vi "Indicate Capillary Line.vi"(8 "error in (no error)":errorcluster, 11 "Capillary in":refnum<class "Capillary.lvclass">) -> (0 "error out":errorcluster, 3 "Capillary out":refnum<class "Capillary.lvclass">)   [LabVIEW 2015, in "AMS UI.lvlib" / "Capillary.lvclass"]
uses:
  Capillary.lvclass
  Capillary.lvclass/Capillary.ctl
  subs/Sample/Sample.lvclass/Sample.ctl
  subs/Sample/Sample.lvclass
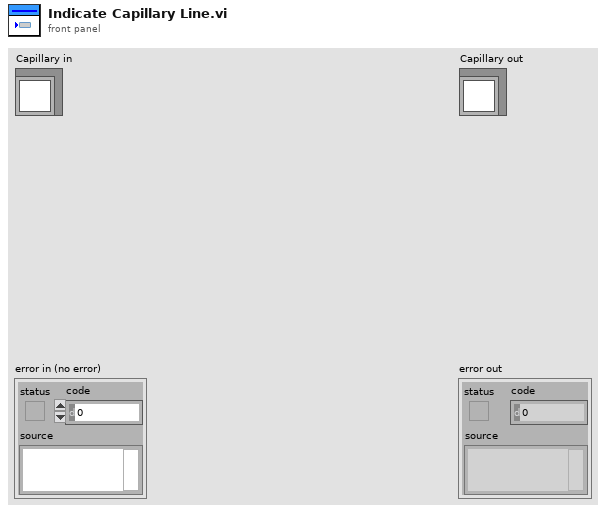
[diagram p1: front panel]
types:
  T1 = typedef "Sample Container.ctl" = cluster{"Sample In":refnum<k21>, "Sample Name":refnum<k21>, "Ti Cathode":refnum<k21>, "SampleQ":refnum<queue>}
  T2 = typedef "FP Control Refs Cluster.ctl" = cluster{"Liquid N Valve References":T3, "Main Line Valve Refs":T4, "Transfer Line Container":refnum<vi>, "Storage Containers":refnum<vi>[], "Sample Refs":T5, "Syringe Ctrl Refs ":T6, "Baratrons Chart":refnum<vi>, "Capillary Container":refnum<vi>, "Preparation Container":refnum<vi>, "Monkey Mode":refnum<vi>}
  T3 = typedef "Liquid N Valve Ref Cluster.ctl" = cluster{"Cold Bath H2O HV 100":refnum<vi>, "Cold Bath Cleaning HV 101":refnum<vi>, "Cold Bath Storage 1 HV 102":refnum<vi>, "Cold Bath Storage 2 HV 103":refnum<vi>, "Cold Bath Storage 3 HV 104":refnum<vi>, "Cold Bath Storage 4 HV 105":refnum<vi>, "Cold Bath Syringe HV 106":refnum<vi>, "Liquid N Master Valve HV 107":refnum<vi>}
  T4 = typedef "Main Line Valve Ref Cluster.ctl" = cluster{"Turbo Valve DV313":refnum<vi>, "Prep Line Valve 0 DV300":refnum<vi>, "Storage Valves":refnum<vi>[]}
  T5 = typedef "Sample Valve Refs.ctl" = cluster{"Valves":cluster{"Sample 5 DV318":refnum<vi>, "Sample 4 DV317":refnum<vi>, "Sample 3 DV316":refnum<vi>, "Sample 2 DV315":refnum<vi>, "Sample 1 DV314":refnum<vi>}, "Lines":cluster{"Sample 1":refnum<vi>, "Sample 2":refnum<vi>, "Sample 3":refnum<vi>, "Sample 4":refnum<vi>, "Sample 5":refnum<vi>}}
  T6 = typedef "Syringe Ctrl Refs.ctl" = cluster{"Syringe Home":refnum<vi>, "Syringe Freeze":refnum<vi>, "Syringe TC":refnum<vi>, "Syringe Container":refnum<vi>}
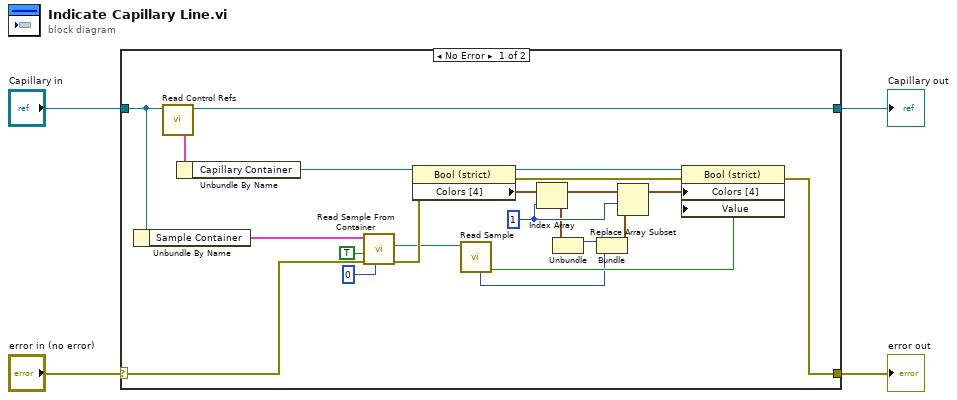
[diagram p0: block diagram]
diagram:
  n1 = case shown="No Error" "error in (no error)" {
    selector: "error in (no error)" -> [w21 w27]
    tunnel: [w5 w27] -> w2
    tunnel: [w25 w26] -> w1
    tunnel: "Capillary in" -> [w23 w26]
    frame No Error {
      w16 = 1 ("index")
      n2 = Unbundle By Name(w23) -> ("Sample Container"=w22:T1)
      n3 = call-dynamic "Read Control Refs.vi"("AMS Gas Actor in"=w23) -> ("Control Refs"=w24:T2, "AMS Gas Actor out"=w25:refnum<class "Capillary.lvclass">)  [unwired: 9 in]
      n4 = Unbundle By Name(w24) -> ("Capillary Container"=w20:refnum<vi>)
      n5 = call "Read Sample From Container.vi"("Queue timeout in ms (-1)"=0, "error in (no error)"=w21, "Read from SHV (F)"=TRUE, "Container"=w22) -> ("error out"=w11:errorcluster, "Sample out"=w10:refnum<class "Sample.lvclass">)  [unwired: 3 in, 3 out]
      n6 = property class="Bool (strict)"(reference=w20, error in=w11) -> (reference out=w19:refnum<vi>, error out=w18:errorcluster, "Colors [4]"=w17:cluster{u32, u32}[])
      n7 = call "Read Sample.vi"("Sample in"=w10) -> ("Sample In"=w9:bool, "Color"=w8:u32)  [unwired: 6 in, 3 out]
      n8 = Index Array(array=w17, index=w16) -> (element=w12:cluster{u32, u32})
      n9 = Unbundle(w12) -> (w13:u32)  [unwired: 1 out]
      n10 = Bundle(w13, "Color"=w8) -> (w15:cluster{u32, "Color":u32})  [unwired: 1 in]
      n11 = Replace Array Subset(array=w17, new element=w15, index=w16) -> (w14:cluster{u32, u32}[])
      n12 = property class="Bool (strict)"(reference=w19, error in=w18, "Colors [4]"=w14, "Value"=w9) -> (error out=w5:errorcluster)  [unwired: 1 out]
    }
    frame Error {
    }
  }
  "error out" <- w2
  "Capillary out" <- w1
